vi "AlliGator Phasor Plot Parameters Scatter Plot.vi"(4 "Time Series Timestamps":dbl[](array[numeric]), 5 "Phasor Plot Idx":i32, 6 "Phasor Frequency":dbl[unit], 7 "Scatter Plot Parameters":T2={"Parameter 2"=enum."Phasor g", "Parameter 1"=enum."Phasor g"}, 8 "error in (no error)":errorcluster, 9 "PhasorPlot Name in":string, 10 "Phasor Plot Data":T1, 11 "AlliGator IV DVR in":refnum<data-value>) -> (0 "error out":errorcluster, 1 "Plot Name out":string, 2 "Parameters Scatter Plot":T1, 3 "AlliGator IV DVR out":refnum<data-value>)   [LabVIEW 2021, in "AlliGator Phasor Graph.lvlib"]
doc: "Computes (P1, P2) scatterplot for the selected Phasor Graph."
uses:
  AlliGator Phasor Graph.lvlib
  Internal Variables/AlliGator Internal Variables v2.ctl
  <vilib>/vision/Image Controls.llb/IMAQ Image.ctl
  Internal Variables/AlliGator Gate Image Set.ctl
  Files/AlliGator FLI Dataset Type.ctl
  Files/AlliGator Data Series Type.ctl
  Dual-Channel Datasets/AlliGator Dataset Channel.ctl
  Settings/AlliGator Gate Arithmetic.ctl
  Source Image/AlliGator Displayed Image.ctl
  Image/Named ROI Description.ctl
  AlliGator Decay Metadata v3.ctl
  Decay Analysis/Decay Preprocessing/AlliGator Decay Background Subtraction Info.ctl
  Decay Analysis/Decay Preprocessing/AlliGator Baseline Subtraction Method.ctl
  Graphs/XY Graph/XY Graph Plot Shift Parameters.ctl
  Graphs/XY Graph/XY Graph Plot Shift Method.ctl
  Decay Analysis/Decay Preprocessing/AlliGator Decay Extrapolation Parameters.ctl
  Phasor/Calibration Phasor (m, phi).ctl
  Phasor/Phasor Reference Series.ctl
  Phasor/Phasor Calibration Map v2.ctl
  Phasor/Phasor (g, s).ctl
  AlliGator Raw Phasor Plot Data v5.ctl
  Phasor/Phasor Standard Deviation Options.ctl
  Phasor Plot/AlliGator Phasor Multi-Harmonic Data.ctl
  Phasor/Phasor Harmonic Data.ctl
  Decay Fit Parameter Map/AlliGator Decay Fit Options & Parameters v3.ctl
  Fits/IRF(X)PSED/Decay Fit Options v3.ctl
  Fits/Decay Convolution/Decay Model.ctl
  Fits/Residual Type.ctl
  Fits/IRF(X)PSED/Fit Weights Type.ctl
  Fits/Non-linear Fitting Method v2.ctl
  Fits/Fit Calculation Method.ctl
  Fits/Non-linear Fitting Algorithm.ctl
  Decay Analysis/Decay Fit/AlliGator Decay Fit Parameter Constraints 2.ctl
  Fits/IRF(X)PSED/Decay Fit Parameters In List.ctl
  Fits/IRF(X)PSED/MLE Baseline Offset Type.ctl
  Decay Analysis/Decay Preprocessing/AlliGator Decay Preprocessing Parameters.ctl
  Fits/IRF(X)PSED/Decay Fit Parameters & Derived Quantities List v2.ctl
  Fits/IRF(X)PSED/Decay Fit Result Constraint.ctl
  Decay Fit Parameter Map/AlliGator Parameter Maps Data.ctl
  Graphs/XY Graph/XY Graph Plot Data.ctl
  AlliGator Phasor Plot Scatter Plot Parameters.ctl
  AlliGator Phasor Graph Parameter List.ctl
  Phasor/Phasor.lvlib
  Image/Image.lvlib
  Decay Analysis/Decay Preprocessing/AlliGator Decay Preprocessing.lvlib
  Files/AlliGator Files.lvlib
  Internal Variables/AlliGator Internal Variables.lvlib
  Phasor Plot/AlliGator Phasor Plot.lvlib
  Source Image/AlliGator Source Image.lvlib
  Fits/Fits.lvlib
  Decay Analysis/Decay Fit/AlliGator Decay Fit.lvlib
  Decay Fit Parameter Map/AlliGator Decay Fit Parameter Map.lvlib
  Settings/AlliGator Settings.lvlib
  Dual-Channel Datasets/AlliGator Dual-Channel Datasets.lvlib
  Graphs/XY Graph/XY Graph Add-Ons.lvlib
panel:
  # "see the AlliGator License on the block diagram (Ctrl+E or Window:Show Block Diagram)"
  # "vs"
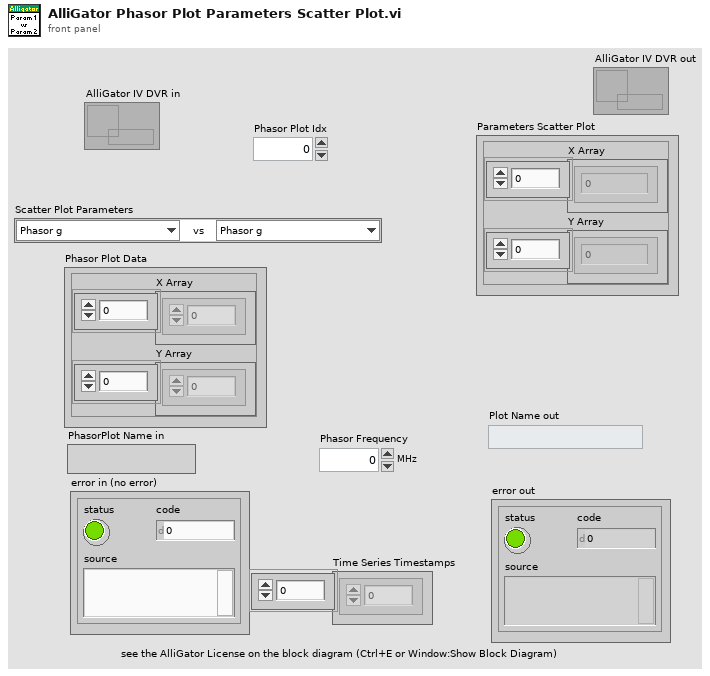
[diagram p1: front panel]
types:
  T1 = typedef "XY Graph Add-Ons.lvlib/XY Graph Plot Data.ctl" = cluster{"X Array":dbl[], "Y Array":dbl[]}
  T2 = typedef "AlliGator Phasor Graph.lvlib/AlliGator Phasor Plot Scatter Plot Parameters.ctl" = cluster{"Parameter 2":T3, "Parameter 1":T3}
  T3 = typedef "AlliGator Phasor Graph.lvlib/AlliGator Phasor Graph Parameter List.ctl" = enum16{"Time Stamp", "Index", "Phasor Parameters", "Phasor g", "Phasor s", "Phasor phi", "Phasor m", "Modulus Lifetime", "Phase Lifetime", "ROI Parameters", "ROI Center x", "ROI Center y", "ROI # pixels ", "Decay Parameters", "Intensity", "Background/Gate", "Intensity - Background", "Fitted Lifetime", "Fitted Intensity", "Phasor Ratio Parameters", "Amplitude Phasor Ratio", "Intensity Phasor Ratio", "Amplitude-Averaged Lifetime", "Intensity-Averaged Lifetime", "-", "Phasor Parameters SDV", "Phasor g SDV", "Phasor s SDV", "Phasor phi SDV", "Phasor m SDV", "Phase Lifetime SDV", "Modulus Lifetime SDV", "Phasor Ratio Parameters SDV", "Amplitude Phasor Ratio SDV", "Intensity Phasor Ratio SDV", "Amplitude-Averaged Lifetime SDV", "Intensity-Averaged Lifetime SDV"}
  T4 = typedef "AlliGator Internal Variables.lvlib/AlliGator Internal Variables v2.ctl" = cluster{"----------------------------- Images -----------------------------":u8, "Displayed Image":T5, "White Light Image":T5, "Mask Image":T5, "ROI Mask Image":T5, "Current Dataset Images 1":T6, "Background Dataset Images 1":T6, "Current Dataset Images 2":T6, "Background Dataset Images 2":T6, "Current Dataset Arithmetic Images":T6, "Accumulated Dataset Images 1":T6, "Accumulated Dataset Images 2":T6, "Accumulated Dataset Arithmetic Images":T6, "----------------------------- File Paths -----------------------------":u8, "Phasor Plot Image":T5, "Decay Fit Parameter Map Image":T5, "Parameter Map Image":T5, "Single Data Point Path":path, "White Light Image Path":path, "Mask Image Path":path, "Time-Series Folder":path, "[Time-Series Paths]":path[], "----------------------------- FLI Dataset -----------------------------":u8, "Current Dataset":i32, "Single Dataset Type":T7, "Current Folder":string, "AlliGator Data Series Type":T8, "# Datasets":i32, "Dual-Channel Dataset":bool, "Selected Channel Name":string, "Dataset Channel":T9, "Channel Arithmetic":T10, "Dual-Channel Background Dataset":bool, "Background Channel":T9, "Dual-Channel Accumulated Dataset":bool, "Start Time":dbl, "[Time-Series Timestamps]":dbl[], "[Intensity Corrections]":dbl[], "Time Series Script":bool, "Type of Displayed Image":T11, "Gate Image Slide":u16, "# Gates":i32, "ROIs":T12[], "----------------------------- Decays -----------------------------":u8, "ROI Decay":cluster{"t Array":dbl[], "I Array":dbl[]}, "Valid Decay":bool, "Decay  Metadata":T14, "Reference Decay Plot Name":string, "Reference Decay":cluster{"t Array":dbl[], "I Array":dbl[]}, "Decay Shift Plot":cluster{"Time Stamps":dbl[], "Decay Shifts":dbl[]}, "[Decays Max Values]":sgl[], "[Decays Min Values]":sgl[], "----------------------------- Calibration -----------------------------":u8, "Calibration Phasor":T20, "Calibration Phasor Series":T21, "Phasor Calibration Map":T22, "Calibration Map MD5 Digest":string, "----------------------------- Phasor Graph -----------------------------":u8, "Last Raw Phasor":T23, "Last Calibrated Phasor":T23, "Last Calibrated Phasor SDV":T23, "Phasor Graph:Phasor Plot":cluster{"g Array":dbl[], "s Array":dbl[]}, "Phasor Graph:Phasor SDV Plot":cluster{"g Array":dbl[], "s Array":dbl[]}, "[Phasor Graph:Raw Phasor Plots]":T24[], "Phasor Plot locked to Ref 1":i32, "[Phasor Plot(s) locked to Ref 1]":i32[], "[Phasor Plot(s) locked to Ref 2]":i32[], "[Pixel Phasors]":T23[], "----------------------------- Phasor Plot -----------------------------":u8, "[[Sum Image]]":dbl[][], "[[CSG Phasors]]":csg[][], "[[Valid Pixel?]]":bool[][], "[[Phasor Ratios]]":dbl[][], "[[Average Lifetimes]]":dbl[][], "Amplitude Weighted Average Lifetime":bool, "I/m/phi Dataset":cluster{"I/m/phi Dataset?":bool, "Base Frequency":dbl[unit], "Harmonic Orders":u8[]}, "Multi Phasor Plot Data":T26, "----------------------------- Decay Fit Parameter Map -----------------------------":u8, "Decay Fit Options & Parameters":T28, "Fit Options: Decay Preprocessing Parameters":T39, "Fit Options: Reference Decay":cluster{"t Array":dbl[], "I Array":dbl[]}, "Is Full Image Parameters Map":bool, "Is Single-Pixels Parameters Map":bool, "NLSF Parameters Map X Resolution":i32, "NLSF Parameters Map Y Resolution":i32, "[Single Decay Fit Parameters]":dbl[], "Fit Model":T30, "[[Multiple Decays Fit Parameters]]":dbl[][], "[[Multiple Decays Fit Parameter SDVs]]":dbl[][], "[[IRFs]]":dbl[][], "IRF Array Time Axis":dbl[], "Decay Array Time Axis":dbl[], "[Decay Fit Parameter Names]":T40[], "[Decay Sum]":dbl[], "Array of Decay Fit Result Constraints":T41[], "Selected ROIs Array":bool[], "----------------------------- Parameter Maps -----------------------------":u8, "[Map Set Names]":string[], "[Parameter Maps]":T42[], "[[User-defined Quantities]]":dbl[][], "User-defined Quantity":string}
  T5 = typedef "IMAQ Image.ctl" = refnum<image>
  T6 = typedef "AlliGator Internal Variables.lvlib/AlliGator Gate Image Set.ctl" = cluster{"SGL Image Max":T5, "SGL Image Sum":T5, "SGL Gate Images":T5[], "SGL Image Min":T5}
  T7 = typedef "AlliGator Files.lvlib/AlliGator FLI Dataset Type.ctl" = enum16{"HDF5 FLI Dataset", "Gate Image Folder", ".sdt FLI Dataset (Becker & Hickl)", ".ptu FLI Dataset (PicoQuant)", "SS1 FLI Dataset", "SS2 FLI Dataset", "I/m/phi Dataset", ".bin FLI Dataset (PicoQuant Binned)", ".bin FLI Dataset (Piccolo Binned)", ".mat FLI Dataset"}
  T8 = typedef "AlliGator Files.lvlib/AlliGator Data Series Type.ctl" = enum16{"Not a Supported Series", "Gate Images Folder Series", "SwissSPAD 2 Dataset Series", "B&H FLI Dataset Series", "PicoQuant PTU FLI Dataset Series", "PicoQuant BIN FLI Dataset Series", "Piccolo hist BIN FLI Dataset Series", "HDF5 FLI Dataset Series"}
  T9 = typedef "AlliGator Dual-Channel Datasets.lvlib/AlliGator Dataset Channel.ctl" = enum16{"G2", "INT"}
  T10 = typedef "AlliGator Settings.lvlib/AlliGator Gate Arithmetic.ctl" = enum16{"None", "INT-G2", "G2/INT*<INT>", "(1 - G2/INT)*<INT>"}
  T11 = typedef "AlliGator Source Image.lvlib/AlliGator Displayed Image.ctl" = enum16{"Single Gate", "Sum of All Gates", "Max of All Gates", "Min of All Gates", "-", "White Ligth Image", "Mask Image"}
  T12 = typedef "Image.lvlib/Named ROI Description.ctl" = cluster{"ROI Descriptor":T13, "ROI Name":string, "Overlay Color":u32}
  T13 = typedef "ROI Descriptor" = cluster{"Global Rectangle":i32[], "Contours":cluster{"ID":enum32{"External", "Internal"}, "Type":u32, "Coordinates":i32[]}[]}
  T14 = typedef "AlliGator Phasor Graph.lvlib/AlliGator Decay Metadata v3.ctl" = cluster{"ROI Descriptor":T13, "ROI Center":cluster{"X":i32, "Y":i32}, "Decay Background Subtraction Info":T15, "Decay Reverted":bool, "Decay Smoothened":bool, "Decay Straightened":bool, "Fitted Tau (Decay Straightening)":dbl, "Decay Shift Parameters":T17, "Decay Shifted":bool, "Decay Extrapolated":bool, "Decay Extrapolation Parameters":T19, "Decay Normalized":bool, "Fold Decay":bool, "# Folds":u32}
  T15 = typedef "AlliGator Decay Preprocessing.lvlib/AlliGator Decay Background Subtraction Info.ctl" = cluster{"Laser Period":dbl[unit], "Gate Duration":dbl[unit], "Baseline Subtraction Method":T16, "Background Definition Range":cluster{"Min Gate":dbl[unit], "Max Gate":dbl[unit]}, "Total Intensity w/o Bkgd Subtraction":dbl, "Bkgd-subtracted Intensity (exp)":dbl, "# Data Points":i32, "Background/Gate":dbl, "Fitted Lifetime":dbl[unit], "Bkgd-subtracted Intensity (theo)":dbl}
  T16 = typedef "AlliGator Decay Preprocessing.lvlib/AlliGator Baseline Subtraction Method.ctl" = enum16{"Mean", "Min", "Square Gated Single-Exponential", "File", "Constant"}
  T17 = typedef "XY Graph Add-Ons.lvlib/XY Graph Plot Shift Parameters.ctl" = cluster{"Type":T18, "Shift":dbl[unit], "Threshold":dbl, "Rotate":bool}
  T18 = typedef "XY Graph Add-Ons.lvlib/XY Graph Plot Shift Method.ctl" = enum16{"Default", "CFD", "Threshold", "Cross-Correlation"}
  T19 = typedef "AlliGator Decay Preprocessing.lvlib/AlliGator Decay Extrapolation Parameters.ctl" = cluster{"Additional Points":u32, "Head Fraction":dbl, "Fitted Tau":dbl, "Use Periodicity":bool, "Use Cursors":bool, "Tail Fraction":dbl}
  T20 = typedef "Phasor.lvlib/Calibration Phasor (m, phi).ctl" = cluster{"m":dbl, "phi":dbl, "Phasor Frequency":dbl[unit], "Reference Lifetime":dbl[unit]}
  T21 = typedef "Phasor.lvlib/Phasor Reference Series.ctl" = cluster{"m Array":dbl[], "phi Array":dbl[], "Phasor Frequency":dbl[unit], "Calibration Lifetime":dbl[unit]}
  T22 = typedef "Phasor.lvlib/Phasor Calibration Map v2.ctl" = cluster{"Phasor Frequency":dbl[unit], "Calibration Lifetime":dbl[unit], "ROI Centers":cluster{"X":i32, "Y":i32}[], "ROI Descriptors":T13[], "Map Resolution X":i32, "Map Resolution Y":i32, "z Array":cdb[]}
  T23 = typedef "Phasor.lvlib/Phasor (g, s).ctl" = cluster{"g":dbl, "s":dbl}
  T24 = typedef "AlliGator Phasor Graph.lvlib/AlliGator Raw Phasor Plot Data v5.ctl" = cluster{"Phasor Plot Name":string, "Raw Phasor Plot":T23[], "Phasor Frequency":dbl[unit], "[Decay Metadata]":T14[], "Raw Phasor Plot SDV":T23[], "Phasor SDV Options":T25, "[Calibration Phasor]":T20[], "Intensity Array":dbl[]}
  T25 = typedef "Phasor.lvlib/Phasor Standard Deviation Options.ctl" = cluster{"Compute Estimated SDV":bool, "# Replicas":u32, "Use Estimated Average Phasor":bool}
  T26 = typedef "AlliGator Phasor Plot.lvlib/AlliGator Phasor Multi-Harmonic Data.ctl" = cluster{"Base Frequency":dbl[unit], "# Harmonics":u8, "Harmonic Orders":u8[], "Phasor Plot Settings Checksum":u64, "Phasor Harmonic Data Array":T27[]}
  T27 = typedef "Phasor.lvlib/Phasor Harmonic Data.ctl" = cluster{"Phasor Harmonic Name":string, "Phasor Plot Settings Checksum":u64, "Phasor Frequency":dbl[unit], "Base Frequency":dbl[unit], "Harmonic Order":u8, "Phasor Plot Parameters":string, "Phasor Array [[CSG]]":csg[][], "Dataset File Path":path}
  T28 = typedef "AlliGator Decay Fit Parameter Map.lvlib/AlliGator Decay Fit Options & Parameters v3.ctl" = cluster{"SYNC Period":dbl[unit], "Fit Options":T29, "Fit Parameter Constraints":T36[], "MLE Baseline Offset":dbl, "MLE Baseline Offset Type":T38}
  T29 = typedef "Fits.lvlib/Decay Fit Options v3.ctl" = cluster{"Show Fit Residuals":bool, "Fit Model":T30, "Residual Type":T31, "Max Decay Percentile":dbl, "Min Decay Percentile":dbl, "Show Full Decay":bool, "Weights":T32, "Fitting Method":T33, "Compute Parameter Uncertainties":bool, "Periodic Boundaries":bool, "Model Calculation":T34, "Period":dbl[unit], "Termination Criteria":cluster{"Max Iterations":i32, "Max Function Calls":i32, "Max Time":dbl[unit], "Function Tolerance":dbl, "Parameter Tolerance":dbl, "Gradient Tolerance":dbl, "Min Lambda":dbl, "Max Lambda":dbl, "Initial Tick Count":u32}, "Offset Resolution":dbl[unit], "Use Local IRF":bool, "Fitting Algorithm":T35, "Show Confidence Interval ":bool, "Confidence Level":dbl}
  T30 = typedef "Fits.lvlib/Decay Model.ctl" = enum16{"1-Exponential", "2-Exponentials"}
  T31 = typedef "Fits.lvlib/Residual Type.ctl" = enum16{"Standard", "Normalized", "Reduced"}
  T32 = typedef "Fits.lvlib/Fit Weights Type.ctl" = enum16{"Unweighted", "1/Variance", "Best of All"}
  T33 = typedef "Fits.lvlib/Non-linear Fitting Method v2.ctl" = enum16{"Least Square", "Least Absolute Residual", "Bisquare", "MLE", "-", "Best of All"}
  T34 = typedef "Fits.lvlib/Fit Calculation Method.ctl" = enum16{"Simulation", "Convolution", "Integration"}
  T35 = typedef "Fits.lvlib/Non-linear Fitting Algorithm.ctl" = enum16{"Levenberg-Marquardt", "Trust-Region Dogleg"}
  T36 = typedef "AlliGator Decay Fit.lvlib/AlliGator Decay Fit Parameter Constraints 2.ctl" = cluster{"Fit Parameter":T37, "Min Value":dbl, "Max Value":dbl, "Global":bool, "Used":bool}
  T37 = typedef "Fits.lvlib/Decay Fit Parameters In List.ctl" = enum16{"Offset", "Baseline", "A_1", "tau_1", "A_2", "tau_2"}
  T38 = typedef "Fits.lvlib/MLE Baseline Offset Type.ctl" = enum32{"Absolute", "Percentage"}
  T39 = typedef "AlliGator Decay Preprocessing.lvlib/AlliGator Decay Preprocessing Parameters.ctl" = cluster{"Background Subtraction":bool, "Straighten Decay":bool, "Reverse Gates":bool, "1-Normalized Decay":bool, "Smoothen Decay":bool, "Smoothing Parameter":dbl, "Shift Decay":bool, "Decay Shift Parameters":T17, "Extrapolate Decay":bool, "Additional Points":u32, "Head Fraction":dbl, "Pixel-Normalize Decay":bool, "Use Periodicity":bool, "Use Cursors":bool, "Tail Fraction":dbl, "Use Decay Pre-Processing":bool, "Fold Decay":bool, "# Folds":u32, "[0-1]-Normalized Decay":bool}
  T40 = typedef "Fits.lvlib/Decay Fit Parameters & Derived Quantities List v2.ctl" = enum16{"Offset", "Baseline", "A_1", "tau_1", "A_2", "tau_2", "<tau>_a", "f1_a", "f2_a", "<tau>_i", "f1_i", "f2_i", "-", "R^2", "Chi^2"}
  T41 = typedef "Fits.lvlib/Decay Fit Result Constraint.ctl" = cluster{"Fit Parameter":enum16{"Offset", "Baseline", "A_1", "tau_1", "A_2", "tau_2", "<tau>_a", "f1_a", "f2_a", "<tau>_i", "f1_i", "f2_i", "-", "R^2", "Chi^2", "Max Relative Residual", "<Residual ACF>", "Residual ACF SDV", "tau_2/tau_1"}, "Min Value":dbl, "Max Value":dbl}
  T42 = typedef "AlliGator Decay Fit Parameter Map.lvlib/AlliGator Parameter Maps Data.ctl" = cluster{"Map Set Name":string, "[Parameter Names]":string[], "[[Parameters]]":dbl[][], "[[Parameter SDVs]]":dbl[][], "Decay Array Time Axis":dbl[], "[[IRFs]]":dbl[][], "IRF Array Time Axis":dbl[], "X Resolution":i32, "Y Resolution":i32, "Intensity Array":dbl[]}
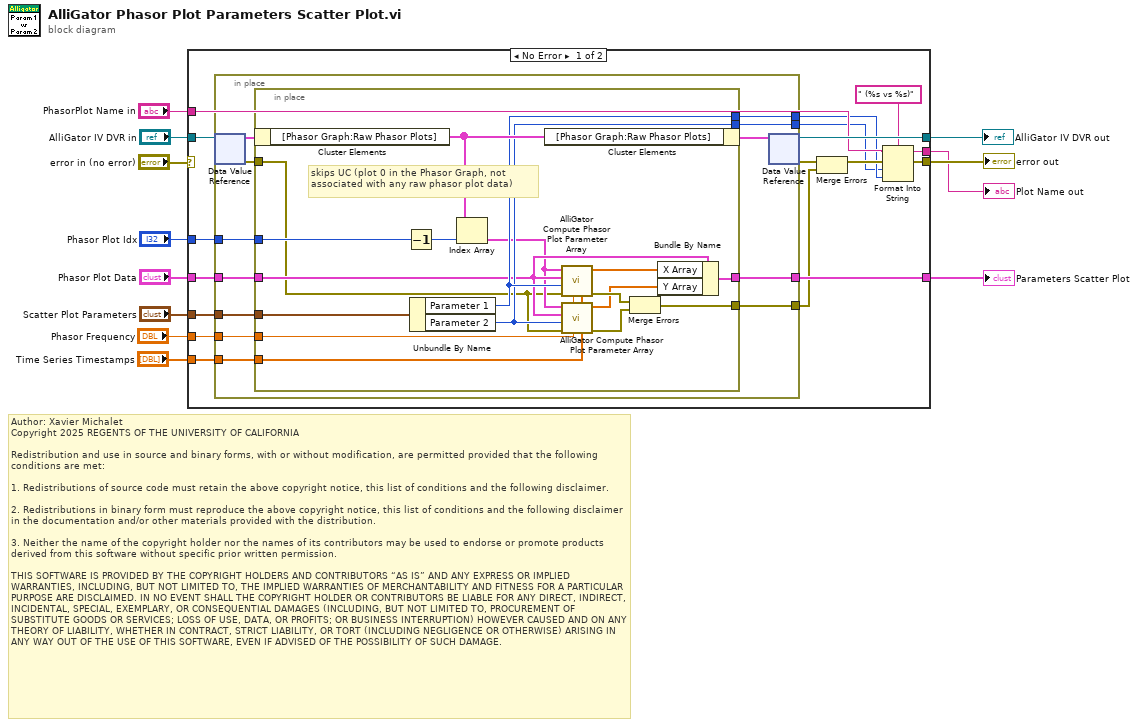
[diagram p0: block diagram]
diagram:
  # "Author: Xavier Michalet\nCopyright 2025 REGENTS OF THE UNIVERSITY OF CALIFORNIA\n\nRedistribution and use in source and binary forms, with or without modification, are permitted provided that the following conditions are met:\n\n1. Redistributions of source code must retain the above copyright notice, this list of conditions and the following disclaimer.\n\n2. Redistributions in binary form must reproduce the above copyright notice, this list of conditions and the following disclaimer in the documentation and/or other materials provided with the distribution.\n\n3. Neither the name of the copyright holder nor the names of its contributors may be used to endorse or promote products derived from this software without specific prior written permission.\n\nTHIS SOFTWARE IS PROVIDED BY THE COPYRIGHT HOLDERS AND CONTRIBUTORS “AS IS” AND ANY EXPRESS OR IMPLIED WARRANTIES, INCLUDING, BUT NOT LIMITED TO, THE IMPLIED WARRANTIES OF MERCHANTABILITY AND FITNESS FOR A PARTICULAR PURPOSE ARE DISCLAIMED. IN NO EVENT SHALL THE COPYRIGHT HOLDER OR CONTRIBUTORS BE LIABLE FOR ANY DIRECT, INDIRECT, INCIDENTAL, SPECIAL, EXEMPLARY, OR CONSEQUENTIAL DAMAGES (INCLUDING, BUT NOT LIMITED TO, PROCUREMENT OF SUBSTITUTE GOODS OR SERVICES; LOSS OF USE, DATA, OR PROFITS; OR BUSINESS INTERRUPTION) HOWEVER CAUSED AND ON ANY THEORY OF LIABILITY, WHETHER IN CONTRACT, STRICT LIABILITY, OR TORT (INCLUDING NEGLIGENCE OR OTHERWISE) ARISING IN ANY WAY OUT OF THE USE OF THIS SOFTWARE, EVEN IF ADVISED OF THE POSSIBILITY OF SUCH DAMAGE."
  n1 = case shown="No Error" "error in (no error)" {
    selector: "error in (no error)" -> [_ w60]
    tunnel: [w29 w59] -> w12
    tunnel: "AlliGator IV DVR in" -> [w28 w59]
    tunnel: [w19 w60] -> w10
    tunnel: "Scatter Plot Parameters" -> [w27 _]
    tunnel: "Phasor Plot Data" -> [w26 _]
    tunnel: [w25 _] -> w6
    tunnel: "Phasor Plot Idx" -> [w24 _]
    tunnel: "Phasor Frequency" -> [w23 _]
    tunnel: "PhasorPlot Name in" -> [w18 _]
    tunnel: [w14 _] -> w2
    tunnel: "Time Series Timestamps" -> [w13 _]
    frame No Error {
      n2 = in-place {
        in-place-border: w27 -> [w39]
        in-place-border: w26 -> [w38]
        in-place-border: [w37] -> w25
        in-place-border: w24 -> [w36]
        in-place-border: w23 -> [w35]
        in-place-border: [w34] -> w21
        in-place-border: [w33] -> w16
        in-place-border: [w32] -> w15
        in-place-border: w13 -> [w30]
        n3 = in-place-dvr #1(w28) -> (w41:T4, w31:errorcluster)
        n4 = in-place {
          in-place-border: w39 -> [w58]
          in-place-border: w38 -> [w48]
          in-place-border: [w56] -> w37
          in-place-border: w36 -> [w54]
          in-place-border: w35 -> [w49]
          in-place-border: [w45] -> w34
          in-place-border: [w51] -> w33
          in-place-border: [w50] -> w32
          in-place-border: w31 -> [w46]
          in-place-border: w30 -> [w42]
          # "skips UC (plot 0 in the Phasor Graph, not associated with any raw phasor plot data)"
          n5 = in-place-cluster #2(w41) -> ("[Phasor Graph:Raw Phasor Plots]"=w55:T24[])
          n6 = Decrement(x=w54) -> (x-1=w53:i32)
          n7 = Unbundle By Name(w58) -> ("Parameter 1"=w51:T3, "Parameter 2"=w50:T3)
          n8 = Index Array(array=w55, index=w53) -> (element=w47:T24)
          n9 = in-place-cluster #2("[Phasor Graph:Raw Phasor Plots]"=w55) -> (w40:T4)
          n10 = call "AlliGator Compute Phasor Plot Parameter Array.vi"("Time Series Timestamps"=w42, "Phasor Frequency"=w49, "error in (no error)"=w46, "Parameter"=w51, "Phasor Plot"=w48, "Raw Phasor Plot"=w47) -> ("error out"=w52:errorcluster, "Parameter Array"=w57:dbl[])  [unwired: 4 in]
          n11 = call "AlliGator Compute Phasor Plot Parameter Array.vi"("Time Series Timestamps"=w42, "Phasor Frequency"=w49, "error in (no error)"=w46, "Parameter"=w50, "Phasor Plot"=w48, "Raw Phasor Plot"=w47) -> ("error out"=w44:errorcluster, "Parameter Array"=w43:dbl[])  [unwired: 4 in]
          n12 = Merge Errors(w52, w44) -> (w45:errorcluster)
          n13 = Bundle By Name(cluster=w48, "X Array"=w57, "Y Array"=w43) -> (w56:T1)
        }
        n14 = in-place-dvr #1(w40) -> (w29:refnum<data-value>, w22:errorcluster)
      }
      n15 = Merge Errors(w22, w21) -> (w20:errorcluster)
      n16 = Format Into String(format string=" (%s vs %s)", initial string=w18, error in=w20, w15, w16) -> (resulting string=w14:string, error out=w19:errorcluster)
    }
    frame Error {
    }
  }
  "error out" <- w10
  "AlliGator IV DVR out" <- w12
  "Parameters Scatter Plot" <- w6
  "Plot Name out" <- w2
